vi "Get TDMS channel info.vi"(8 "error in":errorcluster, 9 "Channel name":string, 10 "group name":string, 11 "tdms file":refnum<k34>) -> (0 "error out":errorcluster, 1 "channel name out":string, 2 "group name out":string, 3 "tdms file out":refnum<k34>, 5 "TDMS channel info":T1)   [LabVIEW 2015]
uses:
  Controls/TDMS channel info.ctl
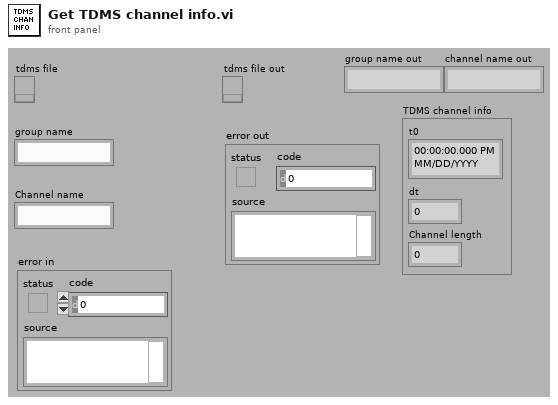
[diagram p1: front panel]
types:
  T1 = typedef "TDMS channel info.ctl" = cluster{"t0":timestamp, "dt":dbl, "Channel length":i64}
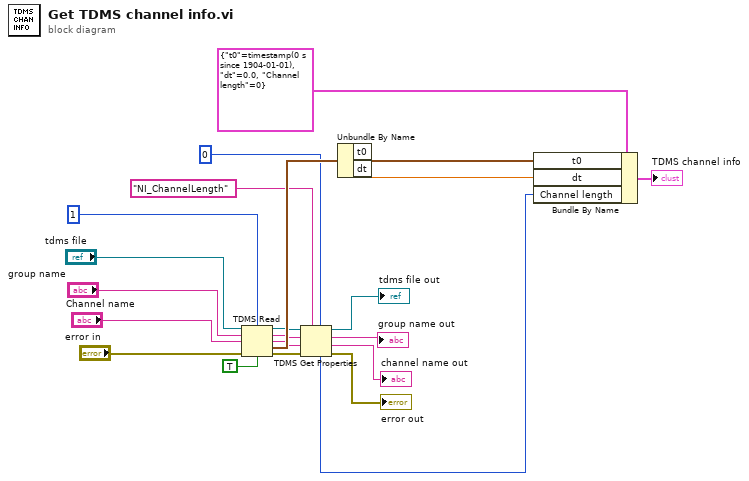
[diagram p0: block diagram]
diagram:
  n1 = TDMS Read(0:"tdms file", 2:i64 1 ("count (-1: all)"), 5:"group name", 7:"Channel name", 11:"error in", 13:TRUE ("return channels in file order? (F)")) -> (4:w15:refnum<k34>, 6:w16:string, 8:w17:string, 10:w18:waveform(dbl), 15:w12:errorcluster)  [unwired: 2 in, 1 out]
  n2 = TDMS Get Properties(5:i64 0, 7:"NI_ChannelLength" ("property name"), 8:w12, 9:w17, 10:w16, 11:w15) -> (0:→"error out":errorcluster, 1:→"channel name out":string, 2:→"group name out":string, 3:→"tdms file out":refnum<k34>, 4:w22:i64)  [unwired: 1 out]
  n3 = Unbundle By Name(w18) -> ("t0"=w20:timestamp, "dt"=w21:dbl)
  n4 = Bundle By Name(cluster=T1 {"t0"=timestamp(0 s since 1904-01-01), "dt"=0.0, "Channel length"=0} ("TDMS channel info"), "t0"=w20, "dt"=w21, "Channel length"=w22) -> (→"TDMS channel info":T1)
